vi "Is 24-bit channel.vi"(5 "DAQmx Physical Channel":tag, 11 "error in (no error)":errorcluster) -> (6 "is 24bit?":bool, 10 "ProductType":string, 15 "error out":errorcluster)   [LabVIEW 2020]
uses:
  <resource>/objmgr/daqmx.rc
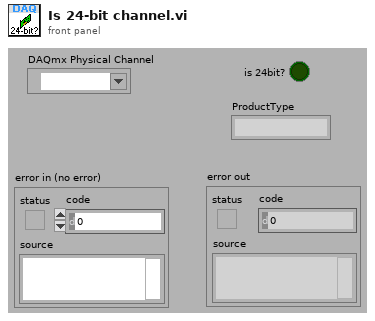
[diagram p1: front panel]
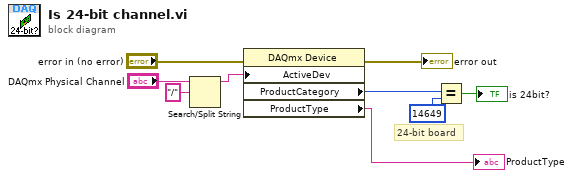
[diagram p0: block diagram]
diagram:
  # "24-bit board"
  n1 = Search/Split String(string="DAQmx Physical Channel", search string/char (-)="/") -> (substring before match=w2:string)  [unwired: 1 in, 2 out]
  n2 = property class="DAQmx Device"(error in="error in (no error)", "ActiveDev"=w2) -> (error out=→"error out":errorcluster, "ProductCategory"=w7:i32, "ProductType"=→"ProductType":string)  [unwired: 1 in, 1 out]
  n3 = Equal?(x=w7, y=14649) -> (x = y?=→"is 24bit?":bool)
